vi "Init Local Reconfig VI.vi"(8 "error in (no error)":errorcluster, 9 "Config Channels":dbl[](array[numeric]), 10 "IOV ref":refnum<k21>, 11 "Module DVR":refnum<data-value>) -> (0 "error out":errorcluster, 3 "Local Reconfig VI Ref":refnum<vi>)   [LabVIEW 2019, in "Scan Engine Custom Device.lvlib"]
uses:
  Scan Engine Custom Device.lvlib
  Modules.lvlibp/RSI Module/RSI Module.lvclass
  Read-Write/Reconfig Local Module.vi
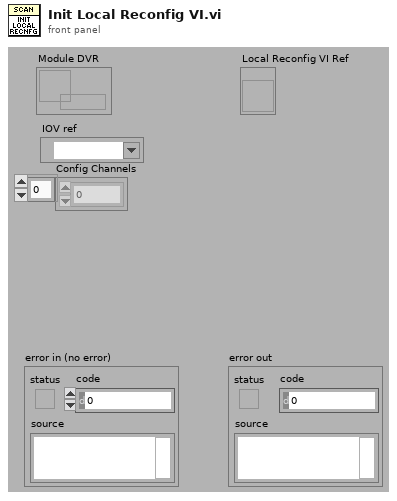
[diagram p1: front panel]
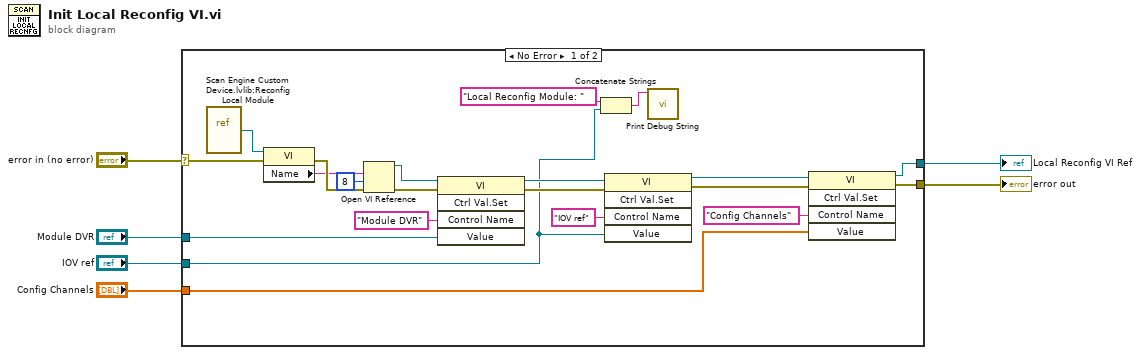
[diagram p0: block diagram]
diagram:
  n1 = case shown="No Error" "error in (no error)" {
    selector: "error in (no error)" -> [w10 w28]
    tunnel: "Module DVR" -> [w27 _]
    tunnel: "IOV ref" -> [w8 _]
    tunnel: "Config Channels" -> [w13 _]
    tunnel: [w12 _] -> w3
    tunnel: [w11 w28] -> w2
    frame No Error {
      n2 = vi-ref "Scan Engine Custom Device.lvlib:Reconfig Local Module.vi"() -> (w24:refnum<vi>)
      n3 = property class="VI"(reference=w24, error in=w10) -> (error out=w25:errorcluster, "Name"=w22:string)  [unwired: 1 out]
      n4 = Open VI Reference(vi path=w22, options=8, error in (no error)=w25) -> (vi reference=w26:refnum<vi>, error out=w23:errorcluster)  [unwired: 3 out]
      n5 = invoke class="VI" method="Ctrl Val.Set"(reference=w26, error in=w23, "Control Name"="Module DVR", "Value"=w27) -> (reference out=w18:refnum<vi>, error out=w17:errorcluster)  [unwired: 1 in, 3 out]
      n6 = Concatenate Strings("Local Reconfig Module: ", w8) -> (w7:string)
      n7 = invoke class="VI" method="Ctrl Val.Set"(reference=w18, error in=w17, "Control Name"="IOV ref", "Value"=w8) -> (reference out=w14:refnum<vi>, error out=w15:errorcluster)  [unwired: 1 in, 3 out]
      n8 = call "Print Debug String.vi"("String to write"=w7) -> ()  [unwired: 9 in, 1 out]
      n9 = invoke class="VI" method="Ctrl Val.Set"(reference=w14, error in=w15, "Control Name"="Config Channels", "Value"=w13) -> (reference out=w12:refnum<vi>, error out=w11:errorcluster)  [unwired: 1 in, 3 out]
    }
    frame Error {
    }
  }
  "Local Reconfig VI Ref" <- w3
  "error out" <- w2
